vi "MoveMeasurement.vi"(10 "Strings []":string[](array[string])) -> (1 "Cancel?":bool, 2 "Segment Out":string)   [LabVIEW 2013, in "main.lvlib"]
uses:
  main.lvlib
panel:
  in  "Cancel":bool
  in  "Save":bool
  in  "Other":string caption="Andet:"
  in  "Segments":u16(ring) items=["Tå", "Ankel", "Over Knæ", "Under Knæ", "Hæl", "Forfod", "Finger", "Andet"]
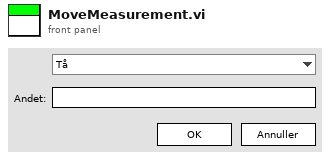
[diagram p1: front panel]
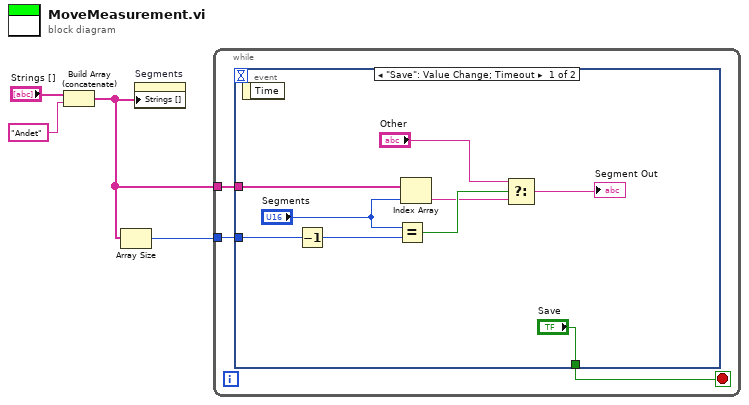
[diagram p0: block diagram]
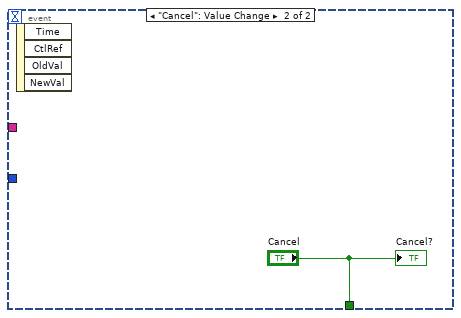
[diagram p2: hidden frame]
diagram:
  n1 = Build Array (concatenate)("Strings []", "Andet") -> (w2:string[])
  n2 = Array Size(array=w2) -> (size(s)=w1:i32)
  n3 = property on="Segments" class="Ring (strict)"("Strings []"=w2) -> ()  [unwired: 2 in, 2 out]
  n4 = while {
    tunnel: w2 -> [w7]
    tunnel: w1 -> [w6]
    stop <- w5 stop-if-true
    n5 = event shown="[0] \"Save\": Value Change;  Timeout" {
      selector: _ -> [_ _]
      dyn-events: _ -> [_ _]
      timeout: _ -> [_ _]
      tunnel: w7 -> [w16 _]
      tunnel: w6 -> [w13 _]
      tunnel: ["Save" "Cancel"] -> w5
      event "Save": Value Change; Timeout {
        n6 = event-data() -> ()  [unwired: 1 in, 1 out]
        n7 = Decrement(x=w13) -> (x-1=w14:i32)
        n8 = Equal?(x="Segments", y=w14) -> (x = y?=w12:bool)
        n9 = Index Array(array=w16, index="Segments") -> (element=w10:string)
        n10 = Select(t="Other", s=w12, f=w10) -> (s? t:f=→"Segment Out":string)
      }
      event "Cancel": Value Change {
        n11 = event-data() -> ()  [unwired: 1 in, 4 out]
        "Cancel?" <- "Cancel"
      }
    }
  }
